vi "Dashboard Main.vi"() -> ()   [LabVIEW 2014]
uses:
  <vilib>/event_ctls.llb/eventvkey.ctl
  <vilib>/Rock Robotics/WPI/Dashboard/WPI_DashboardLogging Global.vi
  <vilib>/Rock Robotics/Network Tables/SD Read Boolean.vi
  <vilib>/Rock Robotics/Network Tables/SD Read Number.vi
  <vilib>/Rock Robotics/Network Tables/SD Write Boolean.vi
  <vilib>/Utility/config.llb/Write Key (String).vi
  <vilib>/Utility/config.llb/Write Key (I32).vi
  <vilib>/Utility/config.llb/NI_LVConfig.lvlib
panel:
  in  "TCP":refnum<k5>
  in  "Rec Mode":enum32{"Stop", "Record", "Playback"}(radio)
  in  "Vision":u16(ring)=1 items=["Camera Off", "USB Camera SW", "USB Camera HW", "IP Camera"]
  out "Camera IP":string
  out "Image Message":string="Timeout in Camera Communications"
  in  "Dashboard Tab":T1(tab)
  in  "Can Left":string(combo)="Can Left"
  out "0":bool
  out "1":bool
  out "2":bool
  out "3":bool
  out "4":bool
  out "5":bool
  out "Fudge Factor":dbl(knob) scale=-100.0..100.0 scale format="%#_4g"
  out "MANUAL":bool
  out "AUTO":bool
  in  "Reset Lift Encoder":bool
  in  "Enable Camera":bool
  in  "Camera Settings":T2={"Frame Rate"=30, "Compression"=30, "Size"=1} {"Frame Rate" scale=1.0..30.0; "Size" items=["640x480", "320x240", "160x120"]}
  out "MotorChart R":cluster{"Numeric":dbl, "Numeric":dbl}(graph)
  out "MotorChart L":T3(graph)
  out "MotorSliders R":cluster{"MotorSlide1":dbl, "MotorSlide2":dbl} {"MotorSlide2" scale=-1.0..1.0 scale format="%#_2e"; "MotorSlide1" scale=-1.0..1.0 scale format="%#_2e"}
  out "MotorSliders L":T4 {"MotorSlide4 2" scale=0.0..14.0 scale format="%#_2e"; "MotorSlide2" scale=-1.0..1.0 scale format="%#_2e"; "MotorSlide1" scale=-1.0..1.0 scale format="%#_2e"}
  out "Gyro":dbl(knob) scale=0.0..360.0
  out "JS1 Z":dbl(slide) scale=-1.0..1.0 scale format="%#_2e"
  out "JS1 Graph":cluster{"X":dbl, "Y":dbl}[](graph)
  out "JS1 Buttons":T5
  out "JS2 Z":dbl(slide) scale=-1.0..1.0 scale format="%#_2e"
  out "JS2 Graph":cluster{"X":dbl, "Y":dbl}[](graph)
  out "JS2 Buttons":T5
  out "Mode":T6(ring)=enum."Auto Disabled"
  in  "DB Camera Config":bool
  out "fps":dbl format="%#.1g"
  out "Mbps":dbl format="%#.1g"
  out "Mbps 2":bool
  in  "DB/String 9":string
  in  "DB/String 8":string
  in  "DB/String 7":string
  in  "DB/String 6":string
  in  "DB/String 5":string
  in  "DB/String 4":string
  in  "DB/String 3":string
  in  "DB/String 2":string
  in  "DB/String 1":string
  in  "DB/String 0":string
  in  "DB/Slider 0":dbl(slide) scale=0.0..5.0
  in  "DB/Slider 1":dbl(slide) scale=0.0..5.0
  in  "DB/Slider 2":dbl(slide) scale=0.0..5.0
  in  "DB/Slider 3":dbl(slide) scale=0.0..5.0
  out "DB/LED 3":bool
  out "DB/LED 2":bool
  out "DB/LED 1":bool
  out "DB/LED 0":bool
  in  "DB/Button 3":bool
  in  "DB/Button 2":bool
  in  "DB/Button 1":bool
  in  "DB/Button 0":bool caption="New Name"
  in  "Test Slider":dbl(slide) scale=0.0..100.0 scale format="%#_3g"
  in  "On/Off":bool caption="Solenoid"
  in  "Test Name":u16(ring) items=["Select the test to run...", "Example Test", "-------------------------------", "List of tests is built in robot code.", "Replace with your own automated tests."]
  in  "Test Tree":string(tree)
  in  "Motor":cluster{"Value":dbl, "Enable":bool} {"Value" scale=-1.0..1.0 scale format="%#_3g"}
  out "Progress":T7 {"Test Progress" scale=0.0..100.0}
  in  "Rev/Fwd":cluster{"Forward":bool, "Reverse":bool}
  in  "Test Ring":u16(ring) items=["Monochrome", "Color"]
  in  "Listbox":i32(listbox)
  out "Tree":string(tree)
  out "Camera Image":T8(plugin-control)
  out "Boolean":bool
  # "L\nI\nF\nT\nE\nR"
  # "Lifter Mode"
  # "L\nE\nV\nE\nL"
  # "Left"
  # "Front"
  # "Right"
  # "Battery"
  # "This tab is a great place for autonomous settings and robot-specific values.\nPlace controls and indicators inside this tab and match name to\nDashboard Variables on robot. You can also delete this comment."
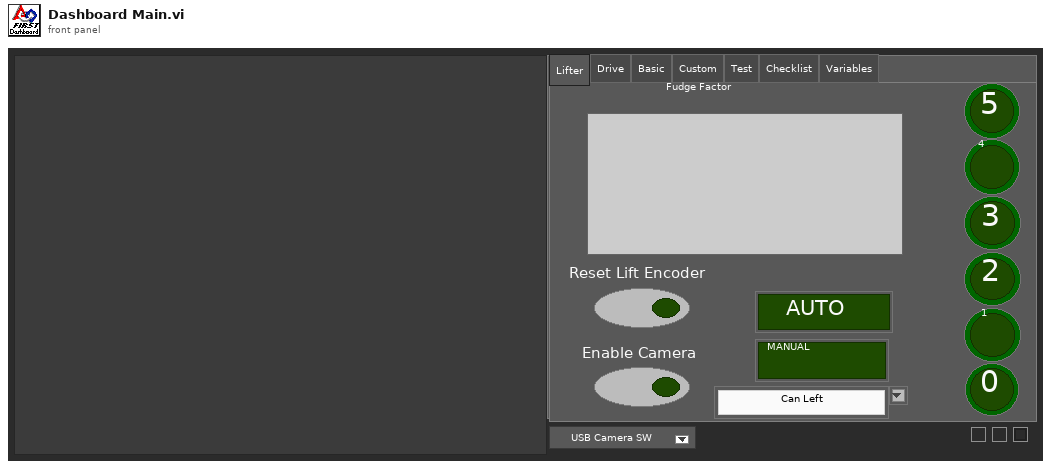
[diagram p1: front panel]
types:
  T1 = enum32{"Lifter", "Drive", "Basic", "Custom", "Test", "Checklist", "Variables"}
  T2 = cluster{"Frame Rate":i32, "Compression":i32, "Size":u16}
  T3 = cluster{"Numeric":dbl, "Numeric":dbl, "Battery V":dbl}
  T4 = cluster{"MotorSlide1":dbl, "MotorSlide2":dbl, "MotorSlide4 2":dbl}
  T5 = cluster{bool, bool, bool, bool, bool, bool, bool, bool, bool, bool, bool, bool}
  T6 = enum8{"Tele-Op Disabled", "Tele-Op Enabled", "Auto Disabled", "Auto Enabled", "Test Disabled", "Test Enabled", "Disconnected", "No Code", "E-Stop"}
  T7 = cluster{"Test Progress":u8, "Test Progress Text":string}
  T8 = typedef "IMAQ Image.ctl" = refnum<image>
  T9 = enum32{"Drive", "Basic", "Custom", "Test", "Checklist", "Variables"}
  T10 = typedef "Image Type" = u32
  T11 = cluster{"Camera Image":refnum<vi>, "Dashboard Tab":refnum<vi>, "Boolean":refnum<vi>, "Vision":refnum<vi>, "Rec Mode":refnum<vi>, "Test Slider":refnum<vi>, "On/Off ":refnum<vi>, "Test Ring":refnum<vi>, "Rev/Fwd":refnum<vi>, "Test Name":refnum<vi>, "Motor":refnum<vi>, "Progress":refnum<vi>, "CheckList":refnum<vi>, "Tree":refnum<vi>, "Test Tree":refnum<vi>}
  T12 = cluster{"Error Strings":string, "Disable Counts":cluster{u16, u16}, "Rail Faults":cluster{u16, u16, u16}, "Robot IP":string, "DB Mode":u8, "Event Info":cluster{"Name":string, "Type":u8, "Number":u16, "Replay":u8}, "Camera Addr":string}
  T13 = cluster{"Storage":cluster{"Disk Free":u64, "RAM Block":u32, "RAM free":u32}, "CPU Utilization":cluster{"CPU % ISR":sgl, "CPU % Time Crit":sgl, "CPU % Timed Str":sgl, "CPU % High":sgl, "CPU % Above":sgl, "CPU % Normal":sgl, "CPU % Low":sgl}, "CAN":cluster{"% Bus Utilization":sgl, "Bus Off Cnt":u32, "TX_FIFO Full Cnt":u32, "Receive Error Cnt":u8, "Transmit Error Cnt":u8}, "HID":cluster{"HID Outputs":u32, "Rumble Low":u16, "Rumble High":u16}[]}
  T14 = cluster{"Status bits":cluster{"Test Mode":bool, "Autonomous":bool, "Enabled":bool, "Code Start":bool, "Brownout":bool, "Reserved 2":bool, "Reserved 3":bool, "E-Stop":bool}, "Code Trace":cluster{"Disabled":bool, "TeleOp":bool, "Auto":bool, "Test":bool}, "Controller Type":enum16{"unknown", "cRIO", "roboRio"}, "Code?":enum16{"unknown", "noCode", "code"}, "Battery V":dbl}
  T15 = cluster{"Control Bits":cluster{"TestMode":bool, "Autonomous":bool, "Enabled":bool, "FMS Present":bool, bool, bool, bool, "E-Stop":bool}, "Team Station ":u8, "Countdown":sgl, "Joystick Values":cluster{"Axes":dbl[], "Buttons":bool[], "POVs":i16[]}[]}
  T16 = cluster{"Axes":dbl[], "Buttons":bool[], "POVs":i16[]}[]
  T17 = cluster{"Axes":dbl[], "Buttons":bool[], "POVs":i16[]}
  T18 = cluster{"Buttons[0]":bool, "Buttons[1]":bool, "Buttons[2]":bool, "Buttons[3]":bool, "Buttons[4]":bool, "Buttons[5]":bool, "Buttons[6]":bool, "Buttons[7]":bool, "Buttons[8]":bool, "Buttons[9]":bool, "Buttons[10]":bool, "Buttons[11]":bool}
  T19 = typedef "NI_LVConfig.lvlib/Config Data RefNum.ctl" = refnum<k1>
  T20 = cluster{"Operation":enum16{"Update", "Clear"}, "Color Box":u32}[]
  T21 = typedef "eventvkey.ctl" = enum16{"ASCII", "Enter", "Return", "Shift", "Ctrl", "Alt", "Cmd", "Opt", "Caps", "NumLock", "Clear", "Break", "Up", "Down", "Left", "Right", "Insert", "Delete", "Home", "End", "PageUp", "PageDown", "Escape", "Help", "Pause", "ScrollLock", "F1", "F2", "F3", "F4", "F5", "F6", "F7", "F8", "F9", "F10", "F11", "F12", "F13", "F14", "F15", "F16", "F17", "F18", "F19", "F20", "F21", "F22", "F23", "F24", "Play", "VolumeUp", "VolumeDown", "Mute", "Two Byte Char"}
  T22 = cluster{"Image Size":bool, "Image Type":bool, "Pixel Value":bool, "ROI Information":bool, "Zoom Factor":bool}
  T23 = enum8{"Enabled", "Disabled", "Disabled and Grayed Out"}
  T24 = cluster{"Operation":enum16{"Update", "Clear"}, "Color Box":u32}
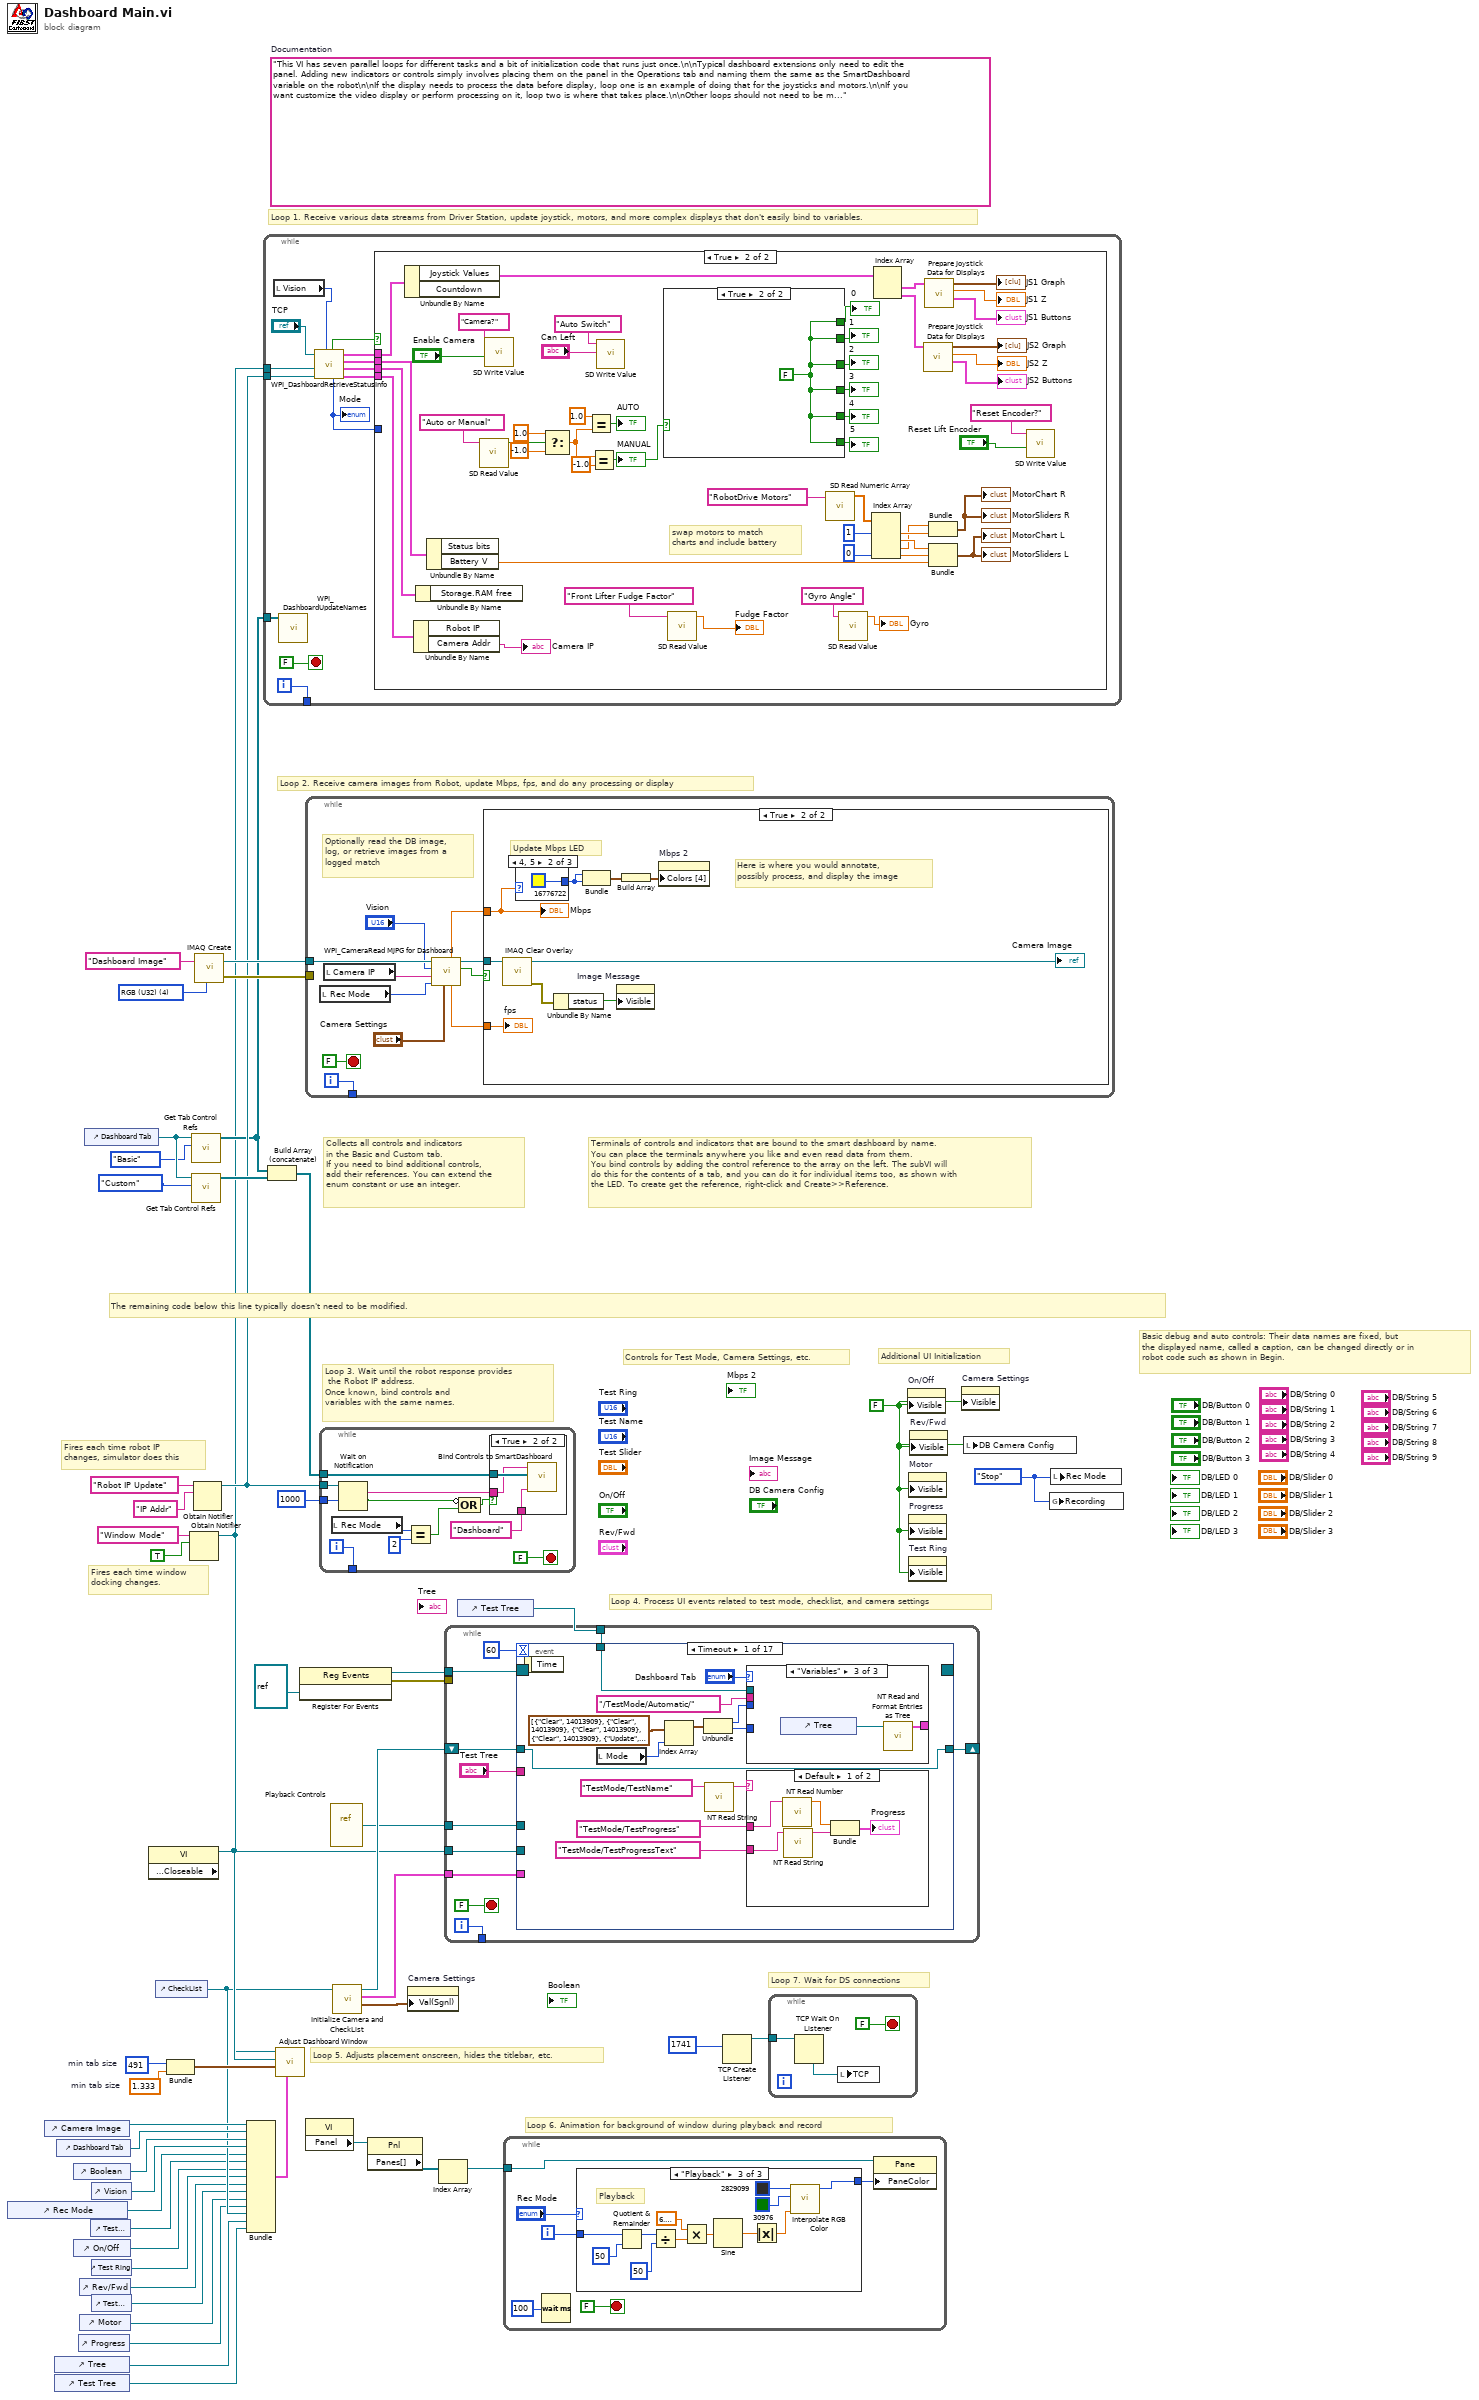
[diagram p0: block diagram]
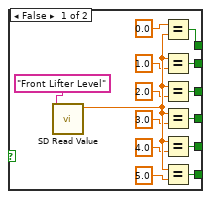
[diagram p3: hidden frame]
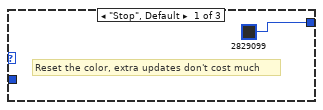
[diagram p4: hidden frame]
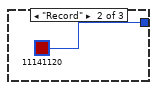
[diagram p5: hidden frame]
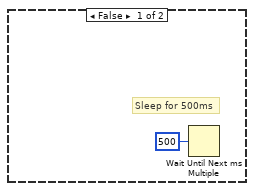
[diagram p7: hidden frame]
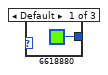
[diagram p8: hidden frame]
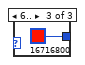
[diagram p9: hidden frame]
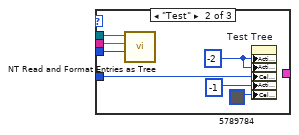
[diagram p11: hidden frame]
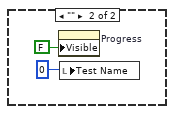
[diagram p12: hidden frame]
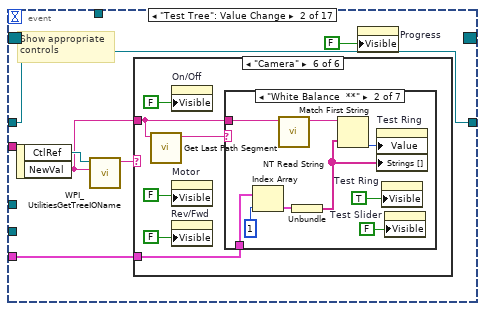
[diagram p13: hidden frame]
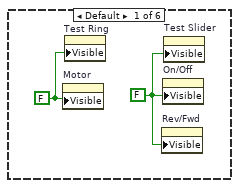
[diagram p14: hidden frame]
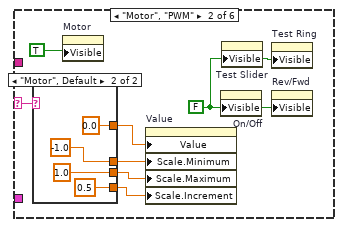
[diagram p15: hidden frame]
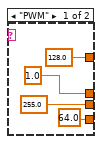
[diagram p16: hidden frame]
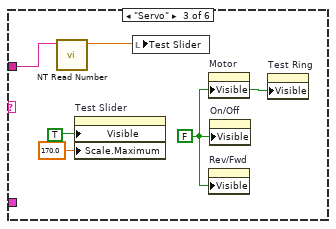
[diagram p17: hidden frame]
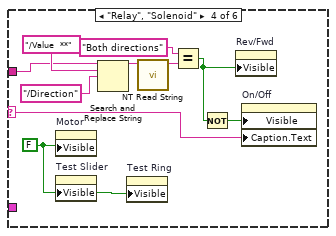
[diagram p18: hidden frame]
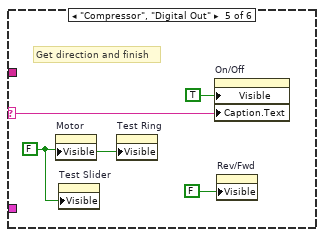
[diagram p19: hidden frame]
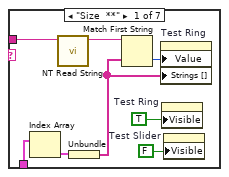
[diagram p20: hidden frame]
diagram:
  w24 = 491  # min tab size
  w23 = 1.333  # min tab size
  w32 = enum32{"Stop", "Record", "Playback"}."Stop" ("Rec Mode")
  w6 = FALSE ("Visible")
  (unwired) "This VI has seven parallel loops for different tasks and a bit of initialization code that runs just once.\n\nTypical dashboard extensions only need to edit the panel. Adding new indicators or controls simply involves placing them on the panel in the Operations tab and naming them the same as the SmartDashboard variable on the robot\n\nIf the display needs to process the data before display, loop one is an example of doing that for the joysticks and motors.\n\nIf you want customize the video display or perform processing on it, loop two is where that takes place.\n\nOther loops should not need to be modified. They are pretty standard, and document the task they perform."  # Documentation
  w52 = T10 4 items=["Grayscale (U8)", "Grayscale (I16)", "Grayscale (SGL)", "Complex (CSG)", "RGB (U32)", "HSL (U32)", "RGB (U64)"] ("Image Type")
  # "Loop 7. Wait for DS connections"
  # "Basic debug and auto controls: Their data names are fixed, but\nthe displayed name, called a caption, can be changed directly or in\nrobot code such as shown in Begin."
  # "Controls for Test Mode, Camera Settings, etc."
  # "Additional UI Initialization"
  # "Loop 6. Animation for background of window during playback and record"
  # "Fires each time robot IP\nchanges, simulator does this"
  # "Fires each time window\ndocking changes."
  # "Collects all controls and indicators\nin the Basic and Custom tab.\nIf you need to bind additional controls,\nadd their references. You can extend the\nenum constant or use an integer."
  # "The remaining code below this line typically doesn't need to be modified."
  # "Loop 4. Process UI events related to test mode, checklist, and camera settings"
  # "Terminals of controls and indicators that are bound to the smart dashboard by name.\nYou can place the terminals anywhere you like and even read data from them.\nYou bind controls by adding the control reference to the array on the left. The subVI will\ndo this for the contents of a tab, and you can do it for individual items too, as shown with\nthe LED. To create get the reference, right-click and Create>>Reference."
  # "Loop 3. Wait until the robot response provides\n the Robot IP address.\nOnce known, bind controls and\nvariables with the same names."
  # "Loop 5. Adjusts placement onscreen, hides the titlebar, etc."
  # "Loop 1. Receive various data streams from Driver Station, update joystick, motors, and more complex displays that don't easily bind to variables."
  # "Loop 2. Receive camera images from Robot, update Mbps, fps, and do any processing or display"
  n1 = control-ref of="Rec Mode"() -> (w12:refnum<vi>)
  n2 = control-ref of="Camera Image"() -> (w27:refnum<vi>)
  n3 = control-ref of="Tree"() -> (w16:refnum<vi>)
  n4 = control-ref of="Test Tree"() -> (w15:refnum<vi>)
  n5 = control-ref of="Dashboard Tab"() -> (w26:refnum<vi>)
  n6 = control-ref of="Boolean"() -> (w21:refnum<vi>)
  n7 = control-ref of="On/Off"() -> (w10:refnum<vi>)
  n8 = control-ref of="Progress"() -> (w7:refnum<vi>)
  n9 = control-ref of="Rev/Fwd"() -> (w8:refnum<vi>)
  n10 = control-ref of="Motor"() -> (w13:refnum<vi>)
  n11 = control-ref of="Dashboard Tab"() -> (w30:refnum<vi>)
  n12 = control-ref of="Test Slider"() -> (w11:refnum<vi>)
  n13 = control-ref of="Vision"() -> (w25:refnum<vi>)
  n14 = control-ref of="Test Ring"() -> (w9:refnum<vi>)
  n15 = control-ref of="Test Name"() -> (w14:refnum<vi>)
  n16 = property class="VI" props=["Front Panel.Closeable"]() -> (reference out=w31:refnum<vi>)  [unwired: 2 in, 2 out]
  n17 = control-ref of="CheckList"() -> (w17:refnum<vi>)
  n18 = Bundle("min tab size"=w24, "min tab size"=w23) -> (w22:cluster{"min tab size":i32, "min tab size":dbl})  [unwired: 1 in]
  n19 = Obtain Notifier(name (unnamed)="Window Mode", notification data type=TRUE) -> (notifier out=w3:refnum<notifier>)  [unwired: 2 in, 2 out]
  n20 = call <vilib>:"Get Tab Control Refs.vi"("Page Index"=T9."Basic" ("Dashboard Tab"), "TabControl in"=w30) -> ("ControlsOnPage"=w4:refnum<vi>[])  [unwired: 9 in]
  n21 = call <vilib>:"Get Tab Control Refs.vi"("Page Index"=T9."Custom" ("Dashboard Tab"), "TabControl in"=w30) -> ("ControlsOnPage"=w29:refnum<vi>[])  [unwired: 9 in]
  n22 = Obtain Notifier(name (unnamed)="Robot IP Update", notification data type="IP Addr" ("name (unnamed)")) -> (notifier out=w5:refnum<notifier>)  [unwired: 2 in, 2 out]
  n23 = call "IMAQ Create"("Image Name"="Dashboard Image", "Image Type"=w52) -> ("New Image"=w50:T8, "error out"=w49:errorcluster)  [unwired: 2 in, 1 out]
  n24 = Bundle("Camera Image"=w27, "Dashboard Tab"=w26, "Boolean"=w21, "Vision"=w25, "Rec Mode"=w12, "Test Slider"=w11, "On/Off"=w10, "Test Ring"=w9, "Rev/Fwd"=w8, "Test Name"=w14, "Motor"=w13, "Progress"=w7, "CheckList"=w17, "Tree"=w16, "Test Tree"=w15) -> (w18:T11)  [unwired: 1 in]
  n25 = while {
    tunnel: [w64] -> _
    tunnel: w5 -> [w58]
    tunnel: w4 -> [w57]
    tunnel: w3 -> [w53]
    i -> [w64]
    stop <- FALSE stop-if-true
    n26 = local read "Vision"() -> (w55:u16)
    n27 = call <vilib>:"WPI_DashboardUpdateNames.vi"("Controls on Tab"=w57) -> ()  [unwired: 11 in]
    n28 = call <vilib>:"WPI_DashboardRetrieveStatusInfo.vi"("Vision"=w55, "Binding Refnum"=w58, "Window Mode Notifier"=w53, "TCP Cnx"="TCP") -> ("Power and Errors"=w59:T12, "Robot Metrics"=w62:T13, "Status Info"=w63:T14, "Control Info"=w60:T15, "Robot Mode"=w56:T6, "Process?"=w61:bool)  [unwired: 2 in]
    "Mode" <- w56
    n29 = case shown="True" w61 {
      tunnel: w63 -> [_ w115]
      tunnel: w62 -> [_ w114]
      tunnel: w60 -> [_ w113]
      tunnel: w59 -> [_ w112]
      tunnel: w56 -> [_ _]
      frame False {
      }
      frame True {
        # "swap motors to match\ncharts and include battery"
        n30 = Unbundle By Name(w113) -> ("Joystick Values"=w100:T16)  [unwired: 1 out]
        n31 = Unbundle By Name(w112) -> ("Camera Addr"=→"Camera IP":string)  [unwired: 1 out]
        n32 = Unbundle By Name(w114) -> ()  [unwired: 1 out]
        n33 = Unbundle By Name(w115) -> ("Battery V"=w101:dbl)  [unwired: 1 out]
        n34 = call-poly <vilib>:"SD Read Value.vi"("Name"="Auto or Manual") -> ("Boolean"=w89:bool)  [unwired: 8 in, 2 out]
        n35 = call-poly <vilib>:"SD Write Value.vi"("Boolean"="Enable Camera", "Name"="Camera?") -> ()  [unwired: 8 in, 2 out]
        n36 = Select(t=1.0, s=w89, f=-1.0) -> (s? t:f=w85:dbl)
        n37 = Equal?(x=1.0, y=w85) -> (x = y?=→"AUTO":bool)
        n38 = Equal?(x=w85, y=-1.0) -> (x = y?=w82:bool)
        "MANUAL" <- w82
        n39 = call-poly <vilib>:"SD Write Value.vi"("Table Prefix"="Can Left", "Name"="Auto Switch") -> ()  [unwired: 8 in, 2 out]
        n40 = case shown="True" w82 {
          tunnel: [w121 w130] -> w81
          tunnel: [w120 w130] -> w80
          tunnel: [w119 w130] -> w79
          tunnel: [w118 w130] -> w78
          tunnel: [w117 w130] -> w77
          tunnel: [w116 w130] -> w76
          frame False {
            n41 = call-poly <vilib>:"SD Read Value.vi"("Name"="Front Lifter Level") -> ("Numeric"=w128:dbl)  [unwired: 8 in, 2 out]
            n42 = Equal?(x=0.0, y=w128) -> (x = y?=w121:bool)
            n43 = Equal?(x=w128, y=1.0) -> (x = y?=w120:bool)
            n44 = Equal?(x=w128, y=2.0) -> (x = y?=w119:bool)
            n45 = Equal?(x=w128, y=3.0) -> (x = y?=w118:bool)
            n46 = Equal?(x=w128, y=4.0) -> (x = y?=w117:bool)
            n47 = Equal?(x=w128, y=5.0) -> (x = y?=w116:bool)
          }
          frame True {
            w130 = FALSE
          }
        }
        "3" <- w78
        "2" <- w79
        "1" <- w80
        "0" <- w81
        "5" <- w76
        "4" <- w77
        n48 = call-poly <vilib>:"SD Read Value.vi"("Name"="Front Lifter Fudge Factor") -> ("Numeric"=→"Fudge Factor":dbl)  [unwired: 8 in, 2 out]
        n49 = call <vilib>:"SD Read Numeric Array.vi"("Name"="RobotDrive Motors") -> ("Numeric Array"=w103:dbl[])  [unwired: 8 in, 2 out]
        n50 = call-poly <vilib>:"SD Read Value.vi"("Name"="Gyro Angle") -> ("Numeric"=→"Gyro":dbl)  [unwired: 8 in, 2 out]
        n51 = Index Array(array=w103, index #1=1, index #4=0) -> (element #1=w107:dbl, element #2=w108:dbl, element #3=w106:dbl, element #4=w111:dbl)  [unwired: 2 in]
        n52 = Index Array(array=w100) -> (element #1=w99:T17, element #2=w94:T17)  [unwired: 2 in]
        n53 = call "Prepare Joystick Data for Displays.vi"("Joystick Values"=w94) -> ("Buttons"=→"JS2 Buttons":T18, "Z Axis"=→"JS2 Z":dbl, "Cartesian Data"=→"JS2 Graph":cluster{"X axis":dbl, "X axis":dbl}[])  [unwired: 8 in]
        n54 = call "Prepare Joystick Data for Displays.vi"("Joystick Values"=w99) -> ("Buttons"=→"JS1 Buttons":T18, "Z Axis"=→"JS1 Z":dbl, "Cartesian Data"=→"JS1 Graph":cluster{"X axis":dbl, "X axis":dbl}[])  [unwired: 8 in]
        n55 = Bundle("Numeric"=w106, "Numeric"=w107) -> (→"MotorChart R" →"MotorSliders R":cluster{"Numeric":dbl, "Numeric":dbl})  [unwired: 1 in]
        n56 = Bundle("Numeric"=w108, "Numeric"=w111, "Battery V"=w101) -> (→"MotorChart L" →"MotorSliders L":T3)  [unwired: 1 in]
        n57 = call-poly <vilib>:"SD Write Value.vi"("Boolean"="Reset Lift Encoder", "Name"="Reset Encoder?") -> ()  [unwired: 8 in, 2 out]
      }
    }
  }
  n58 = Build Array (concatenate)(w4, w29) -> (w28:refnum<vi>[])
  n59 = call "Adjust Dashboard Window.vi"("Sizing Refnums"=w18, "Size Constraints"=w22, "VI"=w31, "Notifier in"=w3) -> ()  [unwired: 8 in]
  n60 = register-events(refnum<vi> refnum) -> (reference out=w36:refnum<event-registration>, error out=w35:errorcluster)  [unwired: 2 in]
  n61 = while {
    tunnel: w50 -> [w139]
    tunnel: w49 -> [_]
    tunnel: [w140] -> _
    i -> [w140]
    stop <- FALSE stop-if-true
    # "Optionally read the DB image,\nlog, or retrieve images from a\nlogged match"
    n62 = local read "Rec Mode"() -> (w133:enum32{"Stop", "Record", "Playback"})
    n63 = local read "Camera IP"() -> (w131:string)
    n64 = call <vilib>:"WPI_CameraRead MJPG for Dashboard.vi"("Camera Settings"="Camera Settings", "Rec Mode"=w133, "Camera IP"=w131, "Camera Mode"="Vision", "Refnum in"=w139) -> ("Active"=w137:bool, "Refnum out"=w138:T8, "FPS"=w136:dbl, "Bandwidth (Mbps)"=w135:dbl)  [unwired: 3 in]
    n65 = case shown="True" w137 {
      tunnel: w138 -> [_ w146]
      tunnel: w135 -> [_ w145]
      tunnel: w136 -> [_ w143]
      frame False {
        # "Sleep for 500ms"
        n66 = Wait Until Next ms Multiple(millisecond multiple=u32 500) -> ()  [unwired: 1 out]
      }
      frame True {
        # "Here is where you would annotate,\npossibly process, and display the image"
        # "Update Mbps LED"
        n67 = call "IMAQ Clear Overlay"("Image"=w146) -> ("error out"=w150:errorcluster, "Image Out"=→"Camera Image":T8)  [unwired: 2 in, 7 out]
        n68 = case shown="4, 5" w145 {
          tunnel: [u32 6618880 ("Color Box") u32 16776722 ("Color Box") u32 16716800 ("Color Box")] -> w147
          frame Default {
          }
          frame 4, 5 {
          }
          frame 6.. {
          }
        }
        n69 = Unbundle By Name(w150) -> ("status"=w151:bool)
        n70 = Bundle("Color Box"=w147, "Color Box"=w147) -> (w149:cluster{"Color Box":u32, "Color Box":u32})  [unwired: 1 out]
        n71 = property on="Image Message" class="Str"("Visible"=w151) -> ()  [unwired: 2 in, 2 out]
        n72 = Build Array(w149) -> (w148:cluster{"Color Box":u32, "Color Box":u32}[])
        n73 = property on="Mbps 2" class="Bool (strict)"("Colors [4]"=w148) -> ()  [unwired: 2 in, 2 out]
        "Mbps" <- w145
        "fps" <- w143
      }
    }
  }
  n74 = property class="VI"() -> ("Panel"=w39:refnum<vi>)  [unwired: 2 in, 2 out]
  n75 = while {
    tunnel: w28 -> [w166]
    tunnel: w5 -> [w164]
    tunnel: [w162] -> _
    tunnel: u32 1000 ("milliseconds to wait") -> [w161]
    i -> [w162]
    stop <- FALSE stop-if-true
    n76 = local read "Rec Mode"() -> (w157:enum32{"Stop", "Record", "Playback"})
    n77 = Wait on Notification(notifier=w164, timeout in ms (-1)=w161) -> (notification=w163:string, timed out?=w159:bool)  [unwired: 2 in, 2 out]
    n78 = Equal?(x=w157, y=u16 2 ("Rec Mode")) -> (x = y?=w158:bool)
    n79 = Compound Arithmetic op=OR(invert w159, w158) -> (w160:bool)
    n80 = case shown="True" w160 {
      tunnel: w166 -> [_ w169]
      tunnel: w163 -> [_ w168]
      tunnel: "Dashboard" -> [_ w167]
      frame False {
      }
      frame True {
        n81 = call <vilib>:"Bind Controls to SmartDashboard.vi"("Client Name"=w167, "Bound Control Refs"=w169, "Server IP Address"=w168) -> ()  [unwired: 9 in]
      }
    }
  }
  n82 = vi-ref "Playback Controls.vi"() -> (w37:refnum<vi>)
  n83 = call "Initialize Camera and CheckList.vi"("ListBox in"=w17) -> ("Cluster"=w43:cluster{"value":i32, "value":i32, "index":i32}, "Array"=w44:cluster{string[]}[], "File Refnum"=w42:T19)  [unwired: 8 in]
  n84 = property class="Pnl"(reference=w39) -> ("Panes[]"=w40:refnum<vi>[])  [unwired: 1 in, 2 out]
  n85 = property on="Camera Settings" class="Clust (strict)"("Val(Sgnl)"=w43) -> ()  [unwired: 2 in, 2 out]
  n86 = Index Array(array=w40) -> (element=w38:refnum<vi>)  [unwired: 1 in]
  n87 = control-ref of="Test Tree"() -> (w41:refnum<vi>)
  n88 = while {
    tunnel: w44 -> [w177]
    shift-right: [w176] -> _
    shift-left: w42 -> [w175]
    tunnel: [w174] -> _
    tunnel: w41 -> [w173]
    tunnel: w37 -> [w172]
    tunnel: w36 -> [w171]
    tunnel: w35 -> [_]
    tunnel: w31 -> [w170]
    i -> [w174]
    stop <- FALSE stop-if-true
    n89 = event shown="[0] Timeout" {
      selector: w171 -> [_ _ _ _ _ _ _ _ _ _ _ _ _ _ _ _ _]
      dyn-events: [_ _ _ _ _ _ _ _ _ _ _ _ _ w415 _ _ _] -> _
      timeout: u32 60 ("milliseconds to wait") -> [_ _ _ _ _ _ _ _ _ _ _ _ _ _ _ _ _]
      tunnel: w173 -> [w189 _ _ _ _ _ _ _ _ _ _ _ _ _ _ _ _]
      tunnel: "Test Tree" -> [_ _ _ _ _ _ _ _ w384 w392 w394 w398 w406 _ _ _ _]
      tunnel: w177 -> [_ w211 _ _ _ _ w348 w378 _ _ _ _ _ _ _ _ _]
      tunnel: [w185 w210 w309 w314 w322 w334 w347 w371 w383 w390 w393 w397 w405 w417 w431 w432 w442] -> w176
      tunnel: w175 -> [w185 w210 w309 w314 w322 w334 w346 w371 w383 w390 w393 w397 w405 w417 w431 w432 w442]
      tunnel: w172 -> [_ _ _ _ _ _ _ _ _ _ _ _ _ w418 _ w435 _]
      tunnel: w170 -> [_ _ _ _ _ _ _ _ _ _ _ _ _ w413 _ _ _]
      event Timeout {
        n90 = event-data() -> ()  [unwired: 1 in, 1 out]
        n91 = local read "Mode"() -> (w188:T6)
        n92 = Index Array(array=T20 [{"Operation"=enum."Clear", "Color Box"=14013909}, {"Operation"=enum."Clear", "Color Box"=14013909}, {"Operation"=enum."Clear", "Color Box"=14013909}, {"Operation"=enum."Clear", "Color Box"=14013909}, {"Operation"=enum."Update", "Color Box"=14013909}, {"Operation"=enum."Update", "Color Box"=16777215}, {"Operation"=enum."Clear", "Color Box"=14013909}, {"Operation"=enum."Clear", "Color Box"=14013909}, {"Operation"=enum."Clear", "Color Box"=14013909}], index=w188) -> (element=w183:T24)
        n93 = Unbundle(w183) -> ("Operation"=w182:enum16{"Update", "Clear"}, "Color Box"=w181:u32)
        n94 = call <vilib>:"NT Read String.vi"("Name"="TestMode/TestName") -> ("String"=w192:string)  [unwired: 9 in, 1 out]
        n95 = case shown="\"Variables\"" "Dashboard Tab" {
          tunnel: w189 -> [_ w200 _]
          tunnel: "/TestMode/Automatic/" ("Name Pattern") -> [_ w199 _]
          tunnel: w182 -> [_ w198 _]
          tunnel: [_ _ w202] -> _
          tunnel: w181 -> [_ w194 _]
          frame "Custom", Default {
          }
          frame "Test" {
            w197 = -2 ("Active Item:Row Number")
            n96 = call <vilib>:"NT Read and Format Entries as Tree.vi"("Operation"=w198, "Name Pattern"=w199, "Tree Refnum"=w200) -> ()  [unwired: 7 in, 2 out]
            n97 = property on="Test Tree" class="Tree (strict)"("Active Item Row Number"=w197, "ActiveColNum"=w197, "CellBG"=w194, "Active Item Row Number"=-1 ("Active Item:Row Number"), "CellBG"=u32 5789784 ("Color Box")) -> ()  [unwired: 2 in, 2 out]
          }
          frame "Variables" {
            n98 = control-ref of="Tree"() -> (w201:refnum<vi>)
            n99 = call <vilib>:"NT Read and Format Entries as Tree.vi"("Tree Refnum"=w201) -> ("Formatted Strings"=w202:cluster{"Name":string, "Value":string}[])  [unwired: 9 in, 1 out]
          }
        }
        n100 = case shown="Default" w192 {
          tunnel: "TestMode/TestProgress" ("Name") -> [w204 _]
          tunnel: "TestMode/TestProgressText" ("Name") -> [w203 _]
          frame Default {
            n101 = call <vilib>:"NT Read Number.vi"("Name"=w204) -> ("Numeric"=w205:dbl)  [unwired: 9 in, 1 out]
            n102 = call <vilib>:"NT Read String.vi"("Name"=w203) -> ("String"=w206:string)  [unwired: 9 in, 1 out]
            n103 = Bundle("Numeric"=w205, "String"=w206) -> (→"Progress":cluster{"Numeric":dbl, "String":string})  [unwired: 1 in]
          }
          frame "" {
            n104 = property on="Progress" class="Clust (strict)"("Visible"=FALSE) -> ()  [unwired: 2 in, 2 out]
            n105 = local write "Test Name"(u16 0) -> ()
          }
        }
      }
      event "Test Tree": Value Change {
        # "Show appropriate\ncontrols"
        n106 = event-data() -> ("CtlRef"=w214:refnum<vi>, "NewVal"=w212:string)  [unwired: 1 in]
        n107 = call <vilib>:"WPI_UtilitiesGetTreeIOName.vi"("NewVal"=w212, "TreeControl in"=w214) -> ("I/O Name"=w215:string)  [unwired: 9 in]
        n108 = case shown="\"Camera\"" w215 {
          selector: w215 -> [_ w222 _ w240 w249 _]
          tunnel: w212 -> [_ _ w237 w239 _ w256]
          tunnel: w211 -> [_ _ _ _ _ w255]
          frame Default {
            w217 = FALSE ("Visible")
            w216 = FALSE ("Visible")
            n109 = property on="Motor" class="Clust (strict)"("Visible"=w216) -> ()  [unwired: 2 in, 2 out]
            n110 = property on="Test Ring" class="Ring (strict)"("Visible"=w216) -> ()  [unwired: 2 in, 2 out]
            n111 = property on="Rev/Fwd" class="Clust (strict)"("Visible"=w217) -> ()  [unwired: 2 in, 2 out]
            n112 = property on="On/Off" class="Bool (strict)"("Visible"=w217) -> ()  [unwired: 2 in, 2 out]
            n113 = property on="Test Slider" class="Slide (strict)"("Visible"=w217) -> ()  [unwired: 2 in, 2 out]
          }
          frame "Motor", "PWM" {
            w223 = FALSE ("Visible")
            n114 = case shown="\"Motor\", Default" w222 {
              tunnel: [1.0 ("Value") -1.0 ("Value")] -> w221
              tunnel: [255.0 ("Value") 1.0 ("Value")] -> w220
              tunnel: [128.0 ("Value") 0.0 ("Value")] -> w219
              tunnel: [64.0 ("Value") 0.5 ("Value")] -> w218
              frame "PWM" {
              }
              frame "Motor", Default {
              }
            }
            n115 = property on="Motor" class="Clust (strict)"("Visible"=TRUE) -> ()  [unwired: 2 in, 2 out]
            n116 = property on="Value" class="Slide (strict)"("Value"=w219, "Scale.Minimum"=w221, "Scale.Maximum"=w220, "Scale.Increment"=w218) -> ()  [unwired: 2 in, 2 out]
            n117 = property on="On/Off" class="Bool (strict)"("Visible"=w223) -> ()  [unwired: 2 in, 2 out]
            n118 = property on="Test Slider" class="Slide (strict)"("Visible"=w223) -> ()  [unwired: 2 in, 2 out]
            n119 = property on="Test Ring" class="Ring (strict)"("Visible"=w223) -> ()  [unwired: 2 in, 2 out]
            n120 = property on="Rev/Fwd" class="Clust (strict)"("Visible"=w223) -> ()  [unwired: 2 in, 2 out]
          }
          frame "Servo" {
            w235 = FALSE ("Visible")
            n121 = call <vilib>:"NT Read Number.vi"("Name"=w237) -> ("Numeric"=w236:dbl)  [unwired: 9 in, 1 out]
            n122 = property on="Test Slider" class="Slide (strict)"("Visible"=TRUE, "Scale.Maximum"=170.0 ("Scale.Range:Maximum")) -> ()  [unwired: 2 in, 2 out]
            n123 = local write "Test Slider"(w236) -> ()
            n124 = property on="Motor" class="Clust (strict)"("Visible"=w235) -> ()  [unwired: 2 in, 2 out]
            n125 = property on="Rev/Fwd" class="Clust (strict)"("Visible"=w235) -> ()  [unwired: 2 in, 2 out]
            n126 = property on="On/Off" class="Bool (strict)"("Visible"=w235) -> ()  [unwired: 2 in, 2 out]
            n127 = property on="Test Ring" class="Ring (strict)"("Visible"=w235) -> ()  [unwired: 2 in, 2 out]
          }
          frame "Relay", "Solenoid" {
            w238 = FALSE ("Visible")
            n128 = property on="Motor" class="Clust (strict)"("Visible"=w238) -> ()  [unwired: 2 in, 2 out]
            n129 = property on="Test Slider" class="Slide (strict)"("Visible"=w238) -> ()  [unwired: 2 in, 2 out]
            n130 = Search and Replace String(input string=w239, search string="/Value  **", replace string="/Direction") -> (result string=w245:string)  [unwired: 5 in, 3 out]
            n131 = property on="Test Ring" class="Ring (strict)"("Visible"=w238) -> ()  [unwired: 2 in, 2 out]
            n132 = call <vilib>:"NT Read String.vi"("Name"=w245) -> ("String"=w243:string)  [unwired: 9 in, 1 out]
            n133 = Equal?(x="Both directions", y=w243) -> (x = y?=w241:bool)
            n134 = Not(x=w241) -> (.not. x?=w242:bool)
            n135 = property on="Rev/Fwd" class="Clust (strict)"("Visible"=w241) -> ()  [unwired: 2 in, 2 out]
            n136 = property on="On/Off" class="Bool (strict)"("Visible"=w242, "Caption.Text"=w240) -> ()  [unwired: 2 in, 2 out]
          }
          frame "Compressor", "Digital Out" {
            w248 = FALSE ("Visible")
            # "Get direction and finish"
            n137 = property on="Motor" class="Clust (strict)"("Visible"=w248) -> ()  [unwired: 2 in, 2 out]
            n138 = property on="Test Slider" class="Slide (strict)"("Visible"=w248) -> ()  [unwired: 2 in, 2 out]
            n139 = property on="Test Ring" class="Ring (strict)"("Visible"=w248) -> ()  [unwired: 2 in, 2 out]
            n140 = property on="On/Off" class="Bool (strict)"("Visible"=TRUE, "Caption.Text"=w249) -> ()  [unwired: 2 in, 2 out]
            n141 = property on="Rev/Fwd" class="Clust (strict)"("Visible"=FALSE) -> ()  [unwired: 2 in, 2 out]
          }
          frame "Camera" {
            n142 = call <vilib>:"Get Last Path Segment.vi"("String in"=w256) -> ("String out"=w257:string)  [unwired: 10 in]
            n143 = property on="On/Off" class="Bool (strict)"("Visible"=FALSE) -> ()  [unwired: 2 in, 2 out]
            n144 = property on="Motor" class="Clust (strict)"("Visible"=FALSE) -> ()  [unwired: 2 in, 2 out]
            n145 = property on="Rev/Fwd" class="Clust (strict)"("Visible"=FALSE) -> ()  [unwired: 2 in, 2 out]
            n146 = case shown="\"White Balance  **\"" w257 {
              tunnel: w256 -> [w263 w272 w281 w290 w299 _ w305]
              tunnel: w255 -> [w261 w269 w278 w287 w296 _ _]
              frame "Size  **" {
                n147 = Index Array(array=w261) -> (element=w260:cluster{string[]})  [unwired: 1 in]
                n148 = call <vilib>:"NT Read String.vi"("Name"=w263) -> ("String"=w262:string)  [unwired: 9 in, 1 out]
                n149 = Unbundle(w260) -> (w258:string[])
                n150 = Match First String(2:w258, 3:w262) -> (0:w259:i32)  [unwired: 1 out]
                n151 = property on="Test Ring" class="Ring (strict)"("Value"=w259, "Strings []"=w258) -> ()  [unwired: 2 in, 2 out]
                n152 = property on="Test Ring" class="Ring (strict)"("Visible"=TRUE) -> ()  [unwired: 2 in, 2 out]
                n153 = property on="Test Slider" class="Slide (strict)"("Visible"=FALSE) -> ()  [unwired: 2 in, 2 out]
              }
              frame "White Balance  **" {
                n154 = Index Array(array=w269, index=1) -> (element=w270:cluster{string[]})
                n155 = call <vilib>:"NT Read String.vi"("Name"=w272) -> ("String"=w271:string)  [unwired: 9 in, 1 out]
                n156 = Unbundle(w270) -> (w267:string[])
                n157 = Match First String(2:w267, 3:w271) -> (0:w266:i32)  [unwired: 1 out]
                n158 = property on="Test Ring" class="Ring (strict)"("Value"=w266, "Strings []"=w267) -> ()  [unwired: 2 in, 2 out]
                n159 = property on="Test Ring" class="Ring (strict)"("Visible"=TRUE) -> ()  [unwired: 2 in, 2 out]
                n160 = property on="Test Slider" class="Slide (strict)"("Visible"=FALSE) -> ()  [unwired: 2 in, 2 out]
              }
              frame "Exposure  **" {
                n161 = Index Array(array=w278, index=2) -> (element=w279:cluster{string[]})
                n162 = call <vilib>:"NT Read String.vi"("Name"=w281) -> ("String"=w280:string)  [unwired: 9 in, 1 out]
                n163 = Unbundle(w279) -> (w275:string[])
                n164 = Match First String(2:w275, 3:w280) -> (0:w276:i32)  [unwired: 1 out]
                n165 = property on="Test Ring" class="Ring (strict)"("Value"=w276, "Strings []"=w275) -> ()  [unwired: 2 in, 2 out]
                n166 = property on="Test Ring" class="Ring (strict)"("Visible"=TRUE) -> ()  [unwired: 2 in, 2 out]
                n167 = property on="Test Slider" class="Slide (strict)"("Visible"=FALSE) -> ()  [unwired: 2 in, 2 out]
              }
              frame "Exposure Priority  **" {
                n168 = Index Array(array=w287, index=3) -> (element=w288:cluster{string[]})
                n169 = call <vilib>:"NT Read String.vi"("Name"=w290) -> ("String"=w289:string)  [unwired: 9 in, 1 out]
                n170 = Unbundle(w288) -> (w284:string[])
                n171 = Match First String(2:w284, 3:w289) -> (0:w285:i32)  [unwired: 1 out]
                n172 = property on="Test Ring" class="Ring (strict)"("Value"=w285, "Strings []"=w284) -> ()  [unwired: 2 in, 2 out]
                n173 = property on="Test Ring" class="Ring (strict)"("Visible"=TRUE) -> ()  [unwired: 2 in, 2 out]
                n174 = property on="Test Slider" class="Slide (strict)"("Visible"=FALSE) -> ()  [unwired: 2 in, 2 out]
              }
              frame "Color Enable  **" {
                n175 = Index Array(array=w296, index=4) -> (element=w297:cluster{string[]})
                n176 = call <vilib>:"NT Read String.vi"("Name"=w299) -> ("String"=w298:string)  [unwired: 9 in, 1 out]
                n177 = Unbundle(w297) -> (w293:string[])
                n178 = Match First String(2:w293, 3:w298) -> (0:w294:i32)  [unwired: 1 out]
                n179 = property on="Test Ring" class="Ring (strict)"("Value"=w294, "Strings []"=w293) -> ()  [unwired: 2 in, 2 out]
                n180 = property on="Test Ring" class="Ring (strict)"("Visible"=TRUE) -> ()  [unwired: 2 in, 2 out]
                n181 = property on="Test Slider" class="Slide (strict)"("Visible"=FALSE) -> ()  [unwired: 2 in, 2 out]
              }
              frame Default {
                n182 = property on="Test Ring" class="Ring (strict)"("Visible"=FALSE) -> ()  [unwired: 2 in, 2 out]
                n183 = property on="Test Slider" class="Slide (strict)"("Visible"=FALSE) -> ()  [unwired: 2 in, 2 out]
              }
              frame "Brightness  **", "Color Level  **", "Compression  **", "FPS  **", "Sharpness  **" {
                n184 = call <vilib>:"NT Read Number.vi"("Name"=w305) -> ("Numeric"=w304:dbl)  [unwired: 9 in, 1 out]
                n185 = local write "Test Slider"(w304) -> ()
                n186 = property on="Test Slider" class="Slide (strict)"("Visible"=TRUE, "Scale.Maximum"=100.0 ("Scale.Range:Maximum")) -> ()  [unwired: 2 in, 2 out]
                n187 = property on="Test Ring" class="Ring (strict)"("Visible"=FALSE) -> ()  [unwired: 2 in, 2 out]
              }
            }
          }
        }
        n188 = property on="Progress" class="Clust (strict)"("Visible"=FALSE) -> ()  [unwired: 2 in, 2 out]
      }
      event "Test Name": Mouse Enter {
        # "Populate the ring with the list of tests"
        n189 = event-data() -> ()  [unwired: 1 in, 1 out]
        n190 = call <vilib>:"NT Read String Array.vi"("Name"="TestMode/TestList") -> ("String Array"=w313:string[])  [unwired: 9 in, 1 out]
        n191 = Build Array (concatenate)("Select the test to run...", w313) -> (w312:string[])
        n192 = property on="Test Name" class="Ring (strict)"("Strings []"=w312) -> ()  [unwired: 2 in, 2 out]
      }
      event "Test Name": Value Change {
        w315 = FALSE ("Visible")
        # "Tell the robot the test name to run"
        n193 = event-data() -> ("NewVal"=w319:u16)  [unwired: 1 in]
        n194 = property on="Test Name" class="Ring (strict)"() -> ("Strings []"=w320:string[])  [unwired: 2 in, 2 out]
        n195 = local write "Progress"(T7 {"Test Progress"=0, "Test Progress Text"=""} ("Progress")) -> ()
        n196 = Index Array(array=w320, index=w319) -> (element=w318:string)
        n197 = call <vilib>:"NT Write String.vi"("String"=w318, "Name"="TestMode/TestName") -> ()  [unwired: 9 in, 1 out]
        n198 = property on="Progress" class="Clust (strict)"("Visible"=TRUE) -> ()  [unwired: 2 in, 2 out]
        n199 = property on="Motor" class="Clust (strict)"("Visible"=w315) -> ()  [unwired: 2 in, 2 out]
        n200 = property on="Test Slider" class="Slide (strict)"("Visible"=w315) -> ()  [unwired: 2 in, 2 out]
        n201 = property on="On/Off" class="Bool (strict)"("Visible"=w315) -> ()  [unwired: 2 in, 2 out]
        n202 = property on="Rev/Fwd" class="Clust (strict)"("Visible"=w315) -> ()  [unwired: 2 in, 2 out]
        n203 = property on="Test Ring" class="Ring (strict)"("Visible"=w315) -> ()  [unwired: 2 in, 2 out]
      }
      event "Listbox": Double Click {
        # "Shift clears all"
        # "Update symbols on the listbox"
        n204 = event-data() -> ("PlatMods.Shift"=w323:bool, "Row"=w325:i32)  [unwired: 1 in]
        n205 = case shown="True" w323 {
          tunnel: w325 -> [w329 _]
          tunnel: 1 -> [w328 _]
          frame False {
            n206 = property on="Listbox" class="LstBox (strict)"() -> ("Item Symbols"=w327:i32[])  [unwired: 2 in, 2 out]
            n207 = Replace Array Subset(array=w327, new element=w328, index=w329) -> (w326:i32[])
            n208 = property on="Listbox" class="LstBox (strict)"("Item Symbols"=w326) -> ()  [unwired: 2 in, 2 out]
          }
          frame True {
            w330 = 0 ("Top Row")
            n209 = property on="Listbox" class="LstBox (strict)"() -> ("Number of Rows"=w332:u32)  [unwired: 2 in, 2 out]
            n210 = Initialize Array(0, w332) -> (w331:i32[])
            n211 = property on="Listbox" class="LstBox (strict)"("Top Row"=w330, "Value"=w330, "Item Symbols"=w331) -> ()  [unwired: 2 in, 2 out]
          }
        }
      }
      event "Listbox": Key Down {
        # "Update symbols on the listbox\nLeft and right keys check and uncheck"
        n212 = event-data() -> ("VKey"=w336:T21)  [unwired: 1 in]
        n213 = case shown="\"Left\", \"Right\"" w336 {
          selector: w336 -> [w341 _]
          tunnel: eventvkey."Left" ("VKey") -> [w339 _]
          frame "Left", "Right" {
            n214 = Equal?(x=w339, y=w341) -> (x = y?=w340:bool)
            n215 = Select(t=0, s=w340, f=1) -> (s? t:f=w342:i32)
            n216 = property on="Listbox" class="LstBox (strict)"() -> ("Item Symbols"=w345:i32[])  [unwired: 2 in, 2 out]
            n217 = Replace Array Subset(array=w345, new element=w342, index="Listbox") -> (w344:i32[])
            n218 = property on="Listbox" class="LstBox (strict)"("Item Symbols"=w344) -> ()  [unwired: 2 in, 2 out]
          }
          frame Default {
          }
        }
      }
      event "DB Camera Config": Value Change {
        # "Show or hide the cluster of controls, store in ini file"
        n219 = event-data() -> ("NewVal"=w349:bool)  [unwired: 1 in]
        n220 = case shown="False" w349 {
          tunnel: w348 -> [w358 _]
          tunnel: [w351 w369] -> w347
          tunnel: w346 -> [w350 w369]
          frame False {
            w365 = "Camera"
            w368 = FALSE ("Visible")
            n221 = local read "Camera Settings"() -> (w357:T2)
            n222 = Index Array(array=w358) -> (element=w361:cluster{string[]})  [unwired: 1 in]
            n223 = Unbundle(w357) -> ("Frame Rate"=w356:i32, "Compression"=w355:i32, "Size"=w359:u16)
            n224 = Unbundle(w361) -> (w360:string[])
            n225 = Index Array(array=w360, index=w359) -> (element=w354:string)
            n226 = call-poly <vilib>:"Write Key.vi"("section"=w365, "value"=w354, "key"="Size", "refnum"=w350) -> ("refnum out"=w367:T19)  [unwired: 2 in, 5 out]
            n227 = call-poly <vilib>:"Write Key.vi"("section"=w365, "value"=w356, "key"="FrameRate", "refnum"=w367) -> ("refnum out"=w366:T19)  [unwired: 1 in, 6 out]
            n228 = property on="Camera Settings" class="Clust (strict)"("Visible"=w368) -> ()  [unwired: 2 in, 2 out]
            n229 = local write "DB Camera Config"(w368) -> ()
            n230 = call-poly <vilib>:"Write Key.vi"("section"=w365, "value"=w355, "key"="Compression", "refnum"=w366) -> ("refnum out"=w352:T19)  [unwired: 1 in, 6 out]
            n231 = call <vilib>:"Close Config Data.vi"("refnum"=w352) -> ("file path"=w353:path)  [unwired: 2 in, 8 out]
            n232 = call <vilib>:"Open Config Data.vi"("configuration file path"=w353) -> ("refnum"=w351:T19)  [unwired: 8 in, 2 out]
          }
          frame True {
            n233 = property on="Camera Settings" class="Clust (strict)"("Visible"=TRUE) -> ()  [unwired: 2 in, 2 out]
          }
        }
      }
      event "Camera Settings": Value Change {
        # "Update summary string when any elements of DB camera change"
        n234 = event-data() -> ("NewVal"=w382:T2)  [unwired: 1 in]
        n235 = Index Array(array=w378) -> (element=w377:cluster{string[]})  [unwired: 1 in]
        n236 = Unbundle(w382) -> ("Frame Rate"=w373:i32, "Compression"=w372:i32, "Size"=w375:u16)
        n237 = Unbundle(w377) -> (w376:string[])
        n238 = Index Array(array=w376, index=w375) -> (element=w374:string)
        n239 = Format Into String(format string="%s   %dfps   %d%%", w374, w373, w372) -> (resulting string=w379:string)  [unwired: 2 in, 1 out]
        n240 = Build Array(w379) -> (w380:string[])
        n241 = property on="DB Camera Config" class="Bool (strict)"("Strings [4]"=w380) -> ()  [unwired: 2 in, 2 out]
      }
      event "Motor.Enable": Value Change {
        # "When the test mode otor enable helper is set, update that\ntree row item's value"
        n242 = event-data() -> ("NewVal"=w388:bool)  [unwired: 1 in]
        n243 = Unbundle("Motor") -> ("Value"=w387:dbl)  [unwired: 1 out]
        n244 = Select(t=w387, s=w388, f=0.0) -> (s? t:f=w385:dbl)
        n245 = call <vilib>:"NT Write Number.vi"("Numeric"=w385, "Name"=w384) -> ()  [unwired: 9 in, 1 out]
      }
      event "Test Slider": Value Change {
        # "When the test mode slider helper is set, update that\ntree row item's value"
        n246 = event-data() -> ("NewVal"=w391:dbl)  [unwired: 1 in]
        n247 = call <vilib>:"NT Write Number.vi"("Numeric"=w391, "Name"=w392) -> ()  [unwired: 9 in, 1 out]
      }
      event "On/Off": Value Change {
        # "When the test mode on/off helper value is set, update that\ntree row item's value"
        n248 = event-data() -> ("NewVal"=w396:bool)  [unwired: 1 in]
        n249 = Boolean To (0,1)(Boolean=w396) -> (0, 1=w395:i16)
        n250 = call <vilib>:"NT Write Number.vi"("Numeric"=w395, "Name"=w394) -> ()  [unwired: 9 in, 1 out]
      }
      event "Rev/Fwd": Value Change {
        # "When the test mode helper value for relays is set, update that\ntree row item's value"
        n251 = event-data() -> ("NewVal.Forward"=w404:bool, "NewVal.Reverse"=w403:bool)  [unwired: 1 in]
        n252 = Boolean To (0,1)(Boolean=w404) -> (0, 1=w400:i16)
        n253 = Boolean To (0,1)(Boolean=w403) -> (0, 1=w402:i16)
        n254 = Negate(x=w402) -> (-x=w401:i16)
        n255 = Add(x=w400, y=w401) -> (x+y=w399:i16)
        n256 = call <vilib>:"NT Write Number.vi"("Numeric"=w399, "Name"=w398) -> ()  [unwired: 9 in, 1 out]
      }
      event "Test Ring": Value Change {
        # "When a test mode helper value is selected from the ring,\nset the tree item's variable to the string value"
        n257 = event-data() -> ("NewVal"=w408:u16)  [unwired: 1 in]
        n258 = property on="Test Ring" class="Ring (strict)"() -> ("Strings []"=w409:string[])  [unwired: 2 in, 2 out]
        n259 = Index Array(array=w409, index=w408) -> (element=w407:string)
        n260 = call <vilib>:"NT Write String.vi"("String"=w407, "Name"=w406) -> ()  [unwired: 9 in, 1 out]
      }
      event "Rec Mode": Value Change {
        # "Update globals for recording mode and path to read log from.\nClear when logging and let NetworkTables set path for vision to\nuse."
        n261 = event-data() -> ("NewVal"=w419:enum32{"Stop", "Record", "Playback"})  [unwired: 1 in]
        n262 = global write "WPI_DashboardLogging Global.vi" "Logging Filename"(path "") -> ()
        n263 = case shown="\"Playback\"" w419 {
          tunnel: w418 -> [_ w421 w429]
          tunnel: [_ _ w428] -> w415
          tunnel: [_ _ w427] -> _
          tunnel: w413 -> [_ _ w425]
          tunnel: cluster{i32, i32} {-250, 170} -> [_ _ w424]
          tunnel: [_ _ T22 {"Image Size"=TRUE, "Image Type"=TRUE, "Pixel Value"=TRUE, "ROI Information"=TRUE, "Zoom Factor"=FALSE} ("Image Information Shown:All Elements")] -> w411
          tunnel: [_ _ TRUE ("Zoom Factor")] -> w410
          frame Default {
          }
          frame "Stop", "Record" {
            # "Place Window too"
            n264 = invoke class="VI" method="FP.Close"(reference=w421) -> (reference out=w420:refnum<vi>)  [unwired: 2 in, 2 out]
            n265 = invoke class="VI" method="Abort VI"(reference=w420) -> ()  [unwired: 2 in, 3 out]
          }
          frame "Playback" {
            n266 = call "Open Playback Panel.vi"("Offset"=w424, "DB VI Ref"=w425, "Playback in"=w429) -> ("Playback out"=w426:refnum<vi>)  [unwired: 8 in]
            n267 = register-events(w426) -> (reference out=w428:refnum<event-registration>, error out=w427:errorcluster)  [unwired: 2 in]
          }
        }
        n268 = global write "WPI_DashboardLogging Global.vi" "Recording"(w419) -> ()
        n269 = property on="Camera Image" class="ImageControl"("Image Information Shown"=w411, "Image Information Visible"=w410) -> ()  [unwired: 2 in, 2 out]
        n270 = call <vilib>:"WPI_DashboardNT Log FieldName Cache.vi"("Operation"=enum16{"Lookup/Add", "Index", "Clear"}."Clear") -> ()  [unwired: 8 in, 3 out]
      }
      event Panel Close {
        w430 = enum32{"Stop", "Record", "Playback"}."Stop" ("Rec Mode")
        # "Playback window has been closed, abort"
        n271 = event-data() -> ()  [unwired: 1 in, 4 out]
        n272 = local write "Rec Mode"(w430) -> ()
        n273 = global write "WPI_DashboardLogging Global.vi" "Recording"(w430) -> ()
      }
      event Panel Close {
        # "Abort playback window and ourself"
        n274 = event-data() -> ()  [unwired: 1 in, 4 out]
        n275 = invoke class="VI" method="FP.Close"(reference=w435) -> (reference out=w434:refnum<vi>)  [unwired: 2 in, 2 out]
        n276 = invoke class="VI" method="Abort VI"(reference=w434) -> (error out=w433:errorcluster)  [unwired: 2 in, 2 out]
        n277 = invoke class="VI" method="Abort VI"(error in=w433) -> ()  [unwired: 2 in, 3 out]
      }
      event "Vision": Value Change {
        # "Enable/Disable Compression slider.\nHW USB is hard-coded into the camera"
        n278 = event-data() -> ("NewVal"=w441:u16)  [unwired: 1 in]
        n279 = Equal?(x=w441, y=u32 2 ("milliseconds to wait")) -> (x = y?=w439:bool)
        n280 = Select(t=T23."Disabled and Grayed Out" ("Disabled"), s=w439, f=T23."Enabled" ("Disabled")) -> (s? t:f=w436:T23)
        n281 = property on="Compression" class="Slide (strict)"("DisabledEnum"=w436) -> ()  [unwired: 2 in, 2 out]
      }
    }
  }
  n282 = while {
    tunnel: w38 -> [w444]
    i -> [w447]
    stop <- FALSE stop-if-true
    n283 = Wait (ms)(milliseconds to wait=u32 100) -> ()  [unwired: 1 out]
    n284 = case shown="\"Playback\"" "Rec Mode" {
      tunnel: w447 -> [_ _ w462]
      tunnel: [u32 2829099 ("Base Color") u32 11141120 ("Target Color") w451] -> w443
      frame "Stop", Default {
        # "Reset the color, extra updates don't cost much"
      }
      frame "Record" {
      }
      frame "Playback" {
        # "Playback"
        n285 = Quotient & Remainder(x=w462, y=u32 50 ("milliseconds to wait")) -> (x-y*floor(x/y)=w458:u32)  [unwired: 1 out]
        n286 = Divide(x=w458, y=u32 50 ("milliseconds to wait")) -> (x/y=w455:dbl)
        n287 = Multiply(x=6.283185307179586, y=w455) -> (x*y=w460:dbl)
        n288 = Sine(x=w460) -> (sin(x)=w459:dbl)
        n289 = Absolute Value(x=w459) -> (abs(x)=w452:dbl)
        n290 = call "Interpolate RGB Color.vi"("Proportion"=w452, "Target Color"=u32 30976, "Base Color"=u32 2829099) -> ("Result Color"=w451:u32)  [unwired: 8 in]
      }
    }
    n291 = property class="Pane"(reference=w444, "PaneColor"=w443) -> ()  [unwired: 1 in, 2 out]
  }
  n292 = TCP Create Listener(10:u16 1741 ("timeout ms (25000)")) -> (3:w1:refnum<k5>)  [unwired: 4 in, 2 out]
  n293 = while {
    tunnel: w1 -> [w464]
    stop <- FALSE stop-if-true
    n294 = TCP Wait On Listener(11:w464) -> (4:w463:refnum<k5>)  [unwired: 3 in, 4 out]
    n295 = local write "TCP"(w463) -> ()
  }
  n296 = property on="On/Off" class="Bool (strict)"("Visible"=w6) -> ()  [unwired: 2 in, 2 out]
  n297 = property on="Motor" class="Clust (strict)"("Visible"=w6) -> ()  [unwired: 2 in, 2 out]
  n298 = property on="Progress" class="Clust (strict)"("Visible"=w6) -> ()  [unwired: 2 in, 2 out]
  n299 = property on="Test Ring" class="Ring (strict)"("Visible"=w6) -> ()  [unwired: 2 in, 2 out]
  n300 = property on="Rev/Fwd" class="Clust (strict)"("Visible"=w6) -> ()  [unwired: 2 in, 2 out]
  n301 = property on="Camera Settings" class="Clust (strict)"("Visible"=w6) -> ()  [unwired: 2 in, 2 out]
  n302 = local write "DB Camera Config"(w6) -> ()
  n303 = global write "WPI_DashboardLogging Global.vi" "Recording"(w32) -> ()
  n304 = local write "Rec Mode"(w32) -> ()
